vi "overlay_landmark_subVI.vi"(6 "Color":u32(colorbox)=16711680, 7 "Group":string, 8 "error in":errorcluster, 9 "Bounding Box":cluster{"x":sgl, "y":sgl}[](array[cluster]), 10 "Position":cluster{"x":sgl, "y":sgl}, 11 "Image":T1) -> (0 "error out":errorcluster, 3 "Image Out":T1)   [LabVIEW 2013]
uses:
  <vilib>/vision/Image Controls.llb/IMAQ Image.ctl
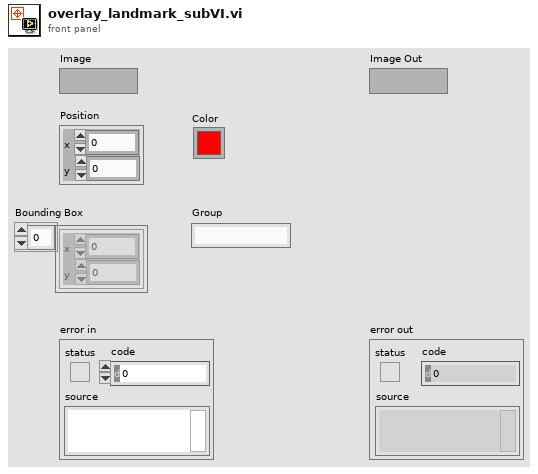
[diagram p1: front panel]
types:
  T1 = typedef "IMAQ Image.ctl" = refnum<image>
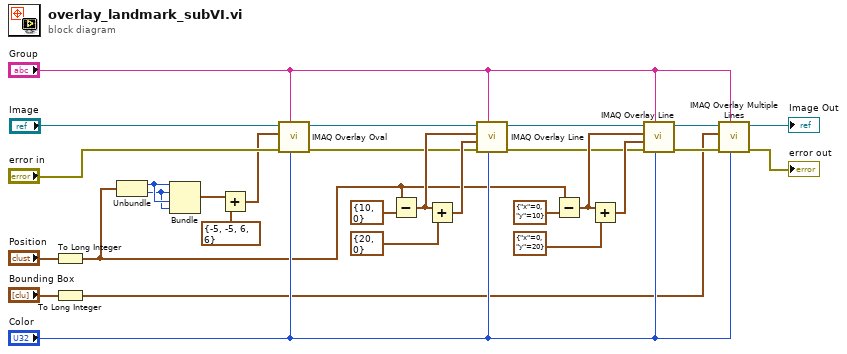
[diagram p0: block diagram]
diagram:
  n1 = To Long Integer(number="Position") -> (32bit integer=w2:cluster{"x":i32, "y":i32})
  n2 = To Long Integer(number="Bounding Box") -> (32bit integer=w1:cluster{"x":i32, "y":i32}[])
  n3 = Unbundle(w2) -> ("x"=w21:i32, "y"=w20:i32)
  n4 = Bundle("x"=w21, "y"=w20, "x"=w21, "y"=w20) -> (w19:cluster{"x":i32, "y":i32, "x":i32, "y":i32})  [unwired: 1 out]
  n5 = Add(x=w19, y=cluster{"y":i32, "x":i32, "y":i32, "x":i32} {"y"=-5, "x"=-5, "y"=6, "x"=6}) -> (x+y=w17:cluster{i32, i32, i32, i32})
  n6 = call "IMAQ Overlay Oval"("Color"="Color", "Group"="Group", "error in (no error)"="error in", "Bounding Rectangle"=w17, "Image"="Image") -> ("error out"=w7:errorcluster, "Image Out"=w23:T1)  [unwired: 1 in, 4 out]
  n7 = Subtract(x=w2, y=cluster{"x":i32, "y":i32} {"x"=10, "y"=0}) -> (x-y=w15:cluster{"x":i32, "y":i32})
  n8 = Add(x=w15, y=cluster{"x":i32, "y":i32} {"x"=20, "y"=0}) -> (x+y=w13:cluster{"x":i32, "y":i32})
  n9 = call "IMAQ Overlay Line"("Color"="Color", "Group"="Group", "error in (no error)"=w7, "End Point"=w13, "Start Point"=w15, "Image"=w23) -> ("error out"=w6:errorcluster, "Image Out"=w8:T1)  [unwired: 4 out]
  n10 = Subtract(x=w2, y=cluster{"x":i32, "y":i32} {"x"=0, "y"=10}) -> (x-y=w11:cluster{"x":i32, "y":i32})
  n11 = Add(x=w11, y=cluster{"x":i32, "y":i32} {"x"=0, "y"=20}) -> (x+y=w12:cluster{"x":i32, "y":i32})
  n12 = call "IMAQ Overlay Line"("Color"="Color", "Group"="Group", "error in (no error)"=w6, "End Point"=w12, "Start Point"=w11, "Image"=w8) -> ("error out"=w5:errorcluster, "Image Out"=w22:T1)  [unwired: 4 out]
  n13 = call "IMAQ Overlay Multiple Lines"("Color"="Color", "Group"="Group", "error in (no error)"=w5, "Line End Points"=w1, "Image"=w22) -> ("error out"=→"error out":errorcluster, "Image Out"=→"Image Out":T1)  [unwired: 1 in, 4 out]
